vi "FPGA_Link.vi"() -> ()   [LabVIEW 2020]
uses:
  <vilib>/Platform/TimedLoop/XDataNode/timing_clust.ctl
  <vilib>/Platform/TimedLoop/XDataNode/nitl_modes.ctl
  <vilib>/Platform/TimedLoop/XDataNode/wakeup.ctl
  <vilib>/rvi/FXPMathLib/basic elements/FxpIntAccumulator/subVIs/nifxpmath_IntAccumulator_SimConfig.ctl
  <vilib>/rvi/Emulation/niFpgaGetClockAttributes.vi
  <vilib>/rvi/Emulation/niFpgaSctlEmulationGetInTimedLoop.vi
  <vilib>/rvi/Emulation/niFpgaEmulationReportErrorSimple.vi
  <vilib>/rvi/eio/common/nirviEmuTemplateMethod_errors.vi
  <vilib>/rvi/Analysis/common/codeGenErrors/XNode/niFpgaXNodeCodeGenErrorHandle.vi
  <vilib>/rvi/Emulation/niFpgaCriticalErrorInLSC.vi
  <vilib>/rvi/FXPMathLib/basic elements/FxpIntAccumulator/simVIs/DllFxpIntAccumulator_sub.vi
  <vilib>/eio/EIONode/EIONode.xnode
  <vilib>/rvi/Analysis/measure/mean-var-std/XNode/niFpgaMean-Var-Std.xnode
  <vilib>/Platform/TimedLoop/XDataNode/XDataNode.xnode
  <vilib>/rvi/FXPMathLib/basic elements/FxpIntAccumulator/XNode/nifxpmath_IntAccumulator.xnode
  <vilib>/rvi/FXPMathLib/FxpMul/XNode/nifxpmath_Multiplier.xnode
  <vilib>/Platform/TimedLoop/XDataNode/XDNodeRunTimeDep.lvlib
  <vilib>/rvi/FXPMathLib/sim/FxpSim.dll
panel:
  in  "Interval":u32=100 caption="Interval(uSec)"
  in  "Swing_Joint_Input":fxp<+/-,20,5>
  in  "Boom_Joint_Input":fxp<+/-,20,5>
  in  "Stick_Joint_Input":fxp<+/-,20,5>
  out "Swing_Joint_Po":fxp<+/-,24,5>
  out "Stick_Joint_Pi":fxp<+/-,48,10>
  out "Boom_Joint_Po":fxp<+/-,24,5>
  out "Boom_Joint_Pi":fxp<+/-,24,5>
  out "Swing_Joint_Pi":fxp<+/-,24,5>
  out "Stick_Joint_Po":fxp<+/-,24,5>
  out "Reference_Pressure":fxp<+/-,24,5>
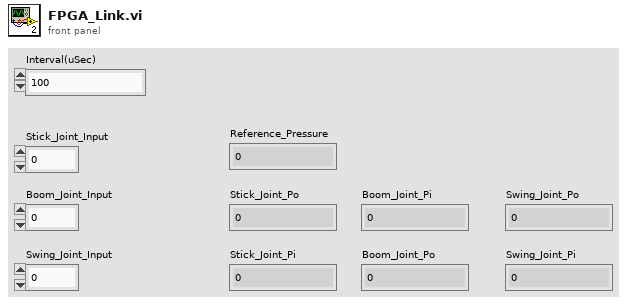
[diagram p1: front panel]
types:
  T1 = typedef "XDNodeRunTimeDep.lvlib/timing_clust.ctl" = cluster{"Expected End [f-1]":u64, "Actual End [f-1]":u64, "Finished Late? [f-1]":bool, "Expected End [i-1]":u64, "Actual End [i-1]":u64, "Finished Late? [i-1]":bool, "Expected Start [i]":u64, "Actual Start [i]":u64, "Expected Start [f]":u64, "Actual Start [f]":u64, "Source Name":string, "Structure Name":string, "Period":i64, "Deadline":i64, "Offset":i64, "Start":i64, "Priority":i32, "Timeout":i32, "Mode":T2, "Wakeup Reason":T3, "Error":errorcluster, "Source Type":string, "Secondary Source Type":string, "Global End Time":u64, "Global Start Time":u64, "Frame Duration":u64, "Iteration Duration":u64, "Assigned CPU":i32, "I/O Scan Engine Mode":u32}
  T2 = typedef "XDNodeRunTimeDep.lvlib/nitl_modes.ctl" = enum32{"No Change", "Process missed periods, maintain original phase", "Discard missed periods, maintain original phase", "Process missed periods, ignore original phase", "Discard missed periods, ignore original phase"}
  T3 = typedef "XDNodeRunTimeDep.lvlib/wakeup.ctl" = enum32{"Normal", "Aborted", "Asynchronous wakeup", "Timing source error", "Timed loop error", "Timeout"}
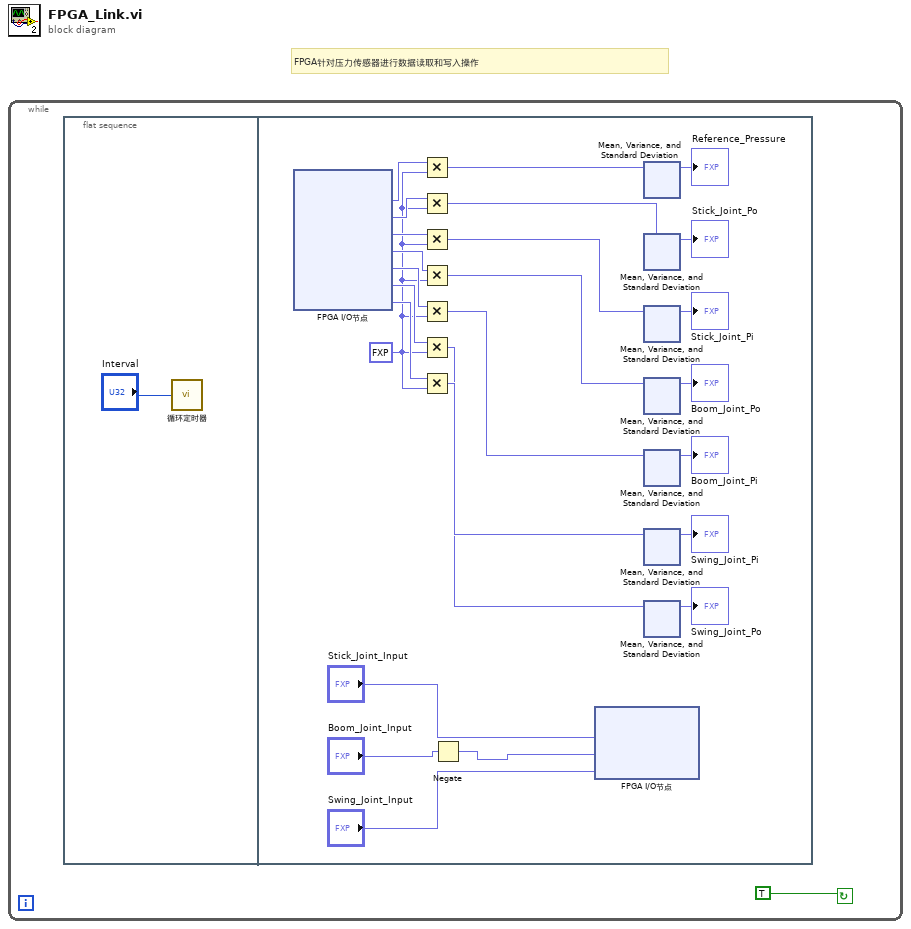
[diagram p0: block diagram]
diagram:
  # "FPGA针对压力传感器进行数据读取和写入操作"
  n1 = while {
    stop <- TRUE continue-if-true
    n2 = flat-sequence {
      frame #0 {
        n3 = call "循环定时器"("Count(uSec)"="Interval") -> ()  [unwired: 1 out]
      }
      frame #1 {
        w17 = fxp<+/-,26,5> 2.5 ("x")
        n4 = xnode "FPGA I/O节点"() -> ("模块1/AI0"=w26:fxp<+/-,24,5>, "模块1/AI1"=w25:fxp<+/-,24,5>, "模块1/AI2"=w24:fxp<+/-,24,5>, "模块1/AI3"=w23:fxp<+/-,24,5>, "模块1/AI4"=w22:fxp<+/-,24,5>, "模块1/AI5"=w21:fxp<+/-,24,5>, "模块1/AI6"=w20:fxp<+/-,24,5>)  [unwired: 7 in, 7 out]
        n5 = Multiply(x=w26, y=w17) -> (x*y=w19:fxp<+/-,50,10>)
        n6 = Multiply(x=w25, y=w17) -> (x*y=w16:fxp<+/-,50,10>)
        n7 = Multiply(x=w24, y=w17) -> (x*y=w14:fxp<+/-,50,10>)
        n8 = Multiply(x=w23, y=w17) -> (x*y=w6:fxp<+/-,50,10>)
        n9 = Multiply(x=w22, y=w17) -> (x*y=w8:fxp<+/-,50,10>)
        n10 = Multiply(x=w21, y=w17) -> (x*y=w10:fxp<+/-,50,10>)
        n11 = Multiply(x=w20, y=w17) -> (x*y=w11:fxp<+/-,50,10>)
        n12 = Negate(x="Boom_Joint_Input") -> (-x=w4:fxp<+/-,21,6>)
        n13 = xnode "FPGA I/O节点"("模块4/AO0"="Stick_Joint_Input", "模块4/AO1"=w4, "模块4/AO2"="Swing_Joint_Input") -> ()  [unwired: 3 in, 3 out]
        n14 = xnode "Mean, Variance, and Standard Deviation"("输入数据"=w19) -> ("均值"=→"Reference_Pressure":fxp<+/-,32,10>)  [unwired: 1 in, 1 out]
        n15 = xnode "Mean, Variance, and Standard Deviation"("输入数据"=w16) -> ("均值"=→"Stick_Joint_Po":fxp<+/-,32,10>)  [unwired: 1 in, 1 out]
        n16 = xnode "Mean, Variance, and Standard Deviation"("输入数据"=w14) -> ("均值"=→"Stick_Joint_Pi":fxp<+/-,32,10>)  [unwired: 1 in, 1 out]
        n17 = xnode "Mean, Variance, and Standard Deviation"("输入数据"=w6) -> ("均值"=→"Boom_Joint_Po":fxp<+/-,32,10>)  [unwired: 1 in, 1 out]
        n18 = xnode "Mean, Variance, and Standard Deviation"("输入数据"=w8) -> ("均值"=→"Boom_Joint_Pi":fxp<+/-,32,10>)  [unwired: 1 in, 1 out]
        n19 = xnode "Mean, Variance, and Standard Deviation"("输入数据"=w11) -> ("均值"=→"Swing_Joint_Pi":fxp<+/-,32,10>)  [unwired: 1 in, 1 out]
        n20 = xnode "Mean, Variance, and Standard Deviation"("输入数据"=w10) -> ("均值"=→"Swing_Joint_Po":fxp<+/-,32,10>)  [unwired: 1 in, 1 out]
      }
    }
  }
